vi "data_acquisition.vi"(11 "error in":errorcluster) -> (4 "output cluster":T1, 15 "error out":errorcluster)   [LabVIEW 2023, in "task_1.lvlib"]
doc: "Generate current and temperature value every 1000 ms"
uses:
  task_1.lvlib
  Data_TC.ctl
  Controls/event_operations.ctl
  Controls/Queue_op.ctl
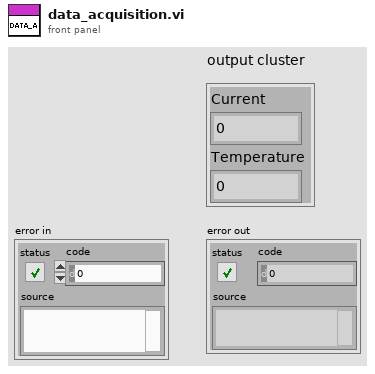
[diagram p1: front panel]
types:
  T1 = typedef "task_1.lvlib/Data_TC.ctl" = cluster{"Current":dbl, "Temperature":dbl}
  T2 = typedef "task_1.lvlib/event_operations.ctl" = enum16{"Create", "Generate", "Get_ref", "Destroy"}
  T3 = typedef "task_1.lvlib/Queue_op.ctl" = enum16{"Create", "Enqueue", "Dequeue", "Destroy"}
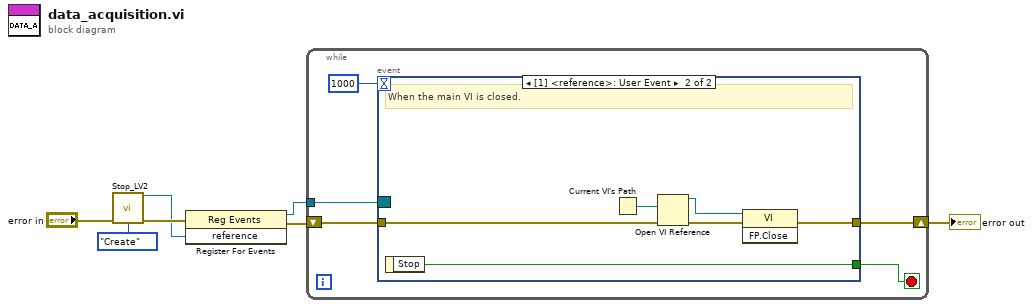
[diagram p0: block diagram]
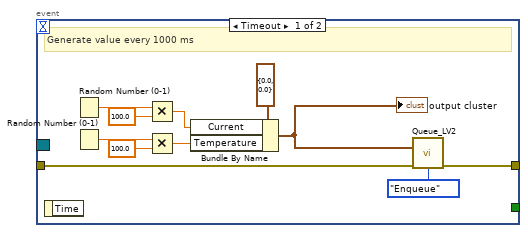
[diagram p2: hidden frame]
diagram:
  n1 = call "Stop_LV2.vi"("error in (no error)"="error in", "Operations"=event_operations."Create") -> ("reference"=w3:refnum<user-event>, "error out"=w5:errorcluster)  [unwired: 12 in]
  n2 = register-events(error in=w5, w3) -> (reference out=w2:refnum<event-registration>, error out=w4:errorcluster)  [unwired: 1 in]
  n3 = while {
    shift-right: [w11] -> w7
    shift-left: w4 -> [w12]
    tunnel: w2 -> [w9]
    stop <- w8 stop-if-true
    n4 = event shown="[1] <reference>: User Event" {
      selector: w9 -> [_ _]
      dyn-events: _ -> [_ _]
      timeout: 1000 -> [_ _]
      tunnel: w12 -> [w15 w28]
      tunnel: [w14 w26] -> w11
      tunnel: [_ w29] -> w8
      event Timeout {
        # "Generate value every 1000 ms"
        n5 = event-data() -> ()  [unwired: 1 in, 1 out]
        n6 = Random Number (0-1)() -> (number: 0 to 1=w23:dbl)
        n7 = Random Number (0-1)() -> (number: 0 to 1=w18:dbl)
        n8 = Multiply(x=w23, y=100.0) -> (x*y=w20:dbl)
        n9 = Multiply(x=w18, y=100.0) -> (x*y=w17:dbl)
        n10 = Bundle By Name(cluster=T1 {"Current"=0.0, "Temperature"=0.0} ("Cluster"), "Current"=w20, "Temperature"=w17) -> (w16:T1)
        "output cluster" <- w16
        n11 = call "Queue_LV2.vi"("element in"=w16, "error in (no error)"=w15, "Operation"=Queue_op."Enqueue") -> ("error IO"=w14:errorcluster)  [unwired: 11 in, 1 out]
      }
      event User Event {
        # "When the main VI is closed."
        n12 = event-data() -> ("Stop"=w29:bool)  [unwired: 1 in]
        n13 = Current VI's Path() -> (path=w24:path)
        n14 = Open VI Reference(vi path=w24, error in (no error)=w28) -> (vi reference=w25:refnum<vi>, error out=w27:errorcluster)  [unwired: 4 in]
        n15 = invoke class="VI" method="FP.Close"(reference=w25, error in=w27) -> (error out=w26:errorcluster)  [unwired: 1 in, 2 out]
      }
    }
  }
  "error out" <- w7
